vi "Balancing Controller.vi"(6 "Configuration":T1={"Accelerometer Bias"={"X (m/s)"=0.0, "Y (m/s)"=0.0, "Z (m/s)"=0.0}, "Gyroscope Bias"={"X (m/s)"=0.0, "Y (m/s)"=0.0, "Z (m/s)"=0.0}, "Steering Motor Gear Ratio"=611.0, "Steering Pully Gear Ratio"=1.0, "Steering Encoder CPR"=500.0, "Steering Motor Max RPM"=4000.0, "Wheelbase (m)"=1.12, "Fork Angle (rad)"=1.3, "Balancing Controller"={"Kp (/s)"=1.0, "Kd (1)"=1.0}, "Max Allowed Steering Angle (rad)"=0.7, "Task Periods"={"Emergency Stop (us)"=10000, "IMU (us)"=10000, "Steering Motor Encoder (us)"=10000, "State Estimator (us)"=10000, "Balancing Controller (us)"=10000, "GNSS (us)"=10000, "Logging (us)"=50000, "Drive Motor (us)"=100000}, "Drive Motor Gear Ratio"=0.7, "lr"=0.4964, "lf"=0.5986, "lambda"=1.2217, "k1"=0.004472, "k2"=0.09678, "e1_max"=11.331, "Ad_t"=0.95971, "Bd_t"=0.01, "C_t"=2.20588, "D_t"=0.0, "Wheel radius"=0.311}, 8 "Measurement In":refnum<data-value>, 9 "State Estimate In":refnum<data-value>, 10 "Trajectory In":refnum<data-value>, 11 "Error In":errorcluster) -> (0 "Measurement Out":refnum<data-value>, 1 "State Estimate Out":refnum<data-value>, 3 "Error Out":errorcluster, 4 "Steering Angle Rate (rad/s)":dbl, 5 "Input balancing":dbl)   [LabVIEW 2021]
uses:
  State Estimator/State Estimate.ctl
  State Estimator/Measurements.ctl
  IMU/IMU Data.ctl
  Steering Motor Encoder/Steering Motor Encoder Data.ctl
  GNSS/GNSS Data.ctl
  Trajectory Control/Trajectory_Control.ctl
  Configuration/Configuration.ctl
  Logging/Log Level.ctl
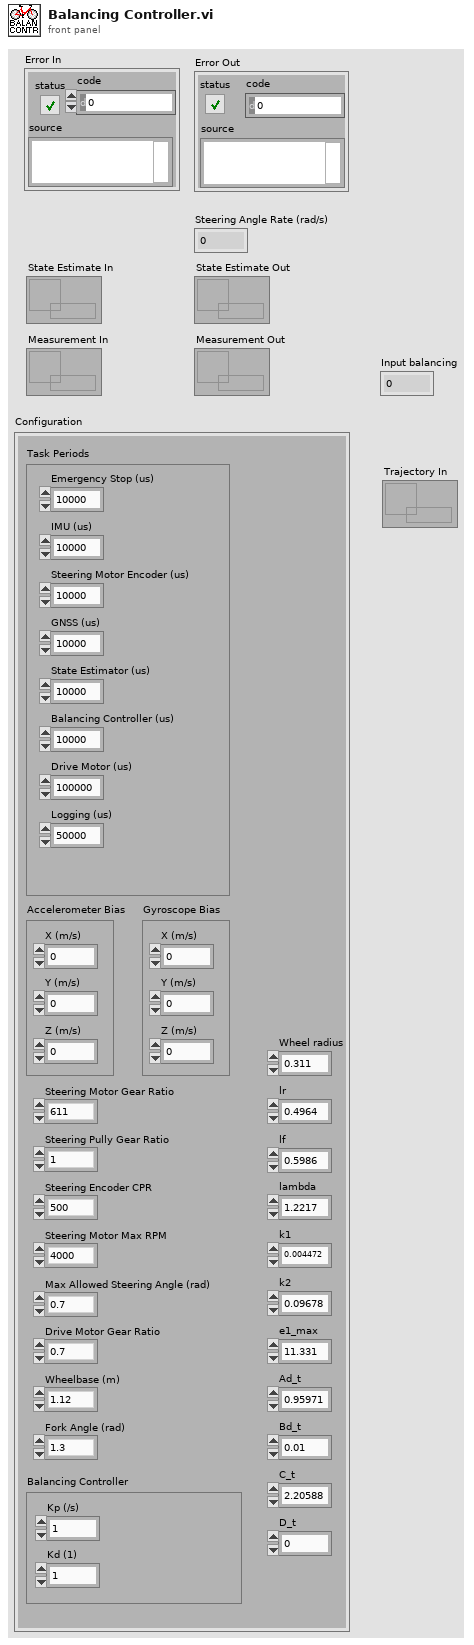
[diagram p1: front panel]
types:
  T1 = typedef "Configuration.ctl" = cluster{"Accelerometer Bias":cluster{"X (m/s)":dbl, "Y (m/s)":dbl, "Z (m/s)":dbl}, "Gyroscope Bias":cluster{"X (m/s)":dbl, "Y (m/s)":dbl, "Z (m/s)":dbl}, "Steering Motor Gear Ratio":dbl, "Steering Pully Gear Ratio":dbl, "Steering Encoder CPR":dbl, "Steering Motor Max RPM":dbl, "Wheelbase (m)":dbl, "Fork Angle (rad)":dbl, "Balancing Controller":cluster{"Kp (/s)":dbl, "Kd (1)":dbl}, "Max Allowed Steering Angle (rad)":dbl, "Task Periods":cluster{"Emergency Stop (us)":i64, "IMU (us)":i64, "Steering Motor Encoder (us)":i64, "State Estimator (us)":i64, "Balancing Controller (us)":i64, "GNSS (us)":i64, "Logging (us)":i64, "Drive Motor (us)":i64}, "Drive Motor Gear Ratio":dbl, "lr":dbl, "lf":dbl, "lambda":dbl, "k1":dbl, "k2":dbl, "e1_max":dbl, "Ad_t":dbl, "Bd_t":dbl, "C_t":dbl, "D_t":dbl, "Wheel radius":dbl}
  T2 = typedef "Log Level.ctl" = enum16{"Error", "Warning", "Info"}
  T3 = typedef "Trajectory_Control.ctl" = cluster{"Rollref":dbl, "Closestpoint":dbl, "Error1":dbl, "Error2":dbl, "Dpsiref_cont":dbl, "Lateral_cont":dbl, "Heading_cont":dbl, "Reset_traj":dbl, "Iteration":dbl}
  T4 = typedef "State Estimate.ctl" = cluster{"X (m)":dbl, "Y (m)":dbl, "Psi (rad)":dbl, "Roll (rad)":dbl, "Roll Rate (rad/s)":dbl, "delta":dbl, "velocity":dbl, "Iterations":dbl}
  T5 = typedef "Measurements.ctl" = cluster{"IMU Data":T6, "Steering Motor Encoder Data":T7, "GNSS Data":T8}
  T6 = typedef "IMU Data.ctl" = cluster{"Gyroscope":cluster{"X (rad/s)":dbl, "Y (rad/s)":dbl, "Z (rad/s)":dbl}, "Accelerometer":cluster{"X (m/s^2)":dbl, "Y (m/s^2)":dbl, "Z (m/s^2)":dbl}, "Flag IMU":dbl}
  T7 = typedef "Steering Motor Encoder Data.ctl" = cluster{"Encoder Position (counts)":i32, "Steering Angle (rad)":dbl, "Flag Steering Encoder":dbl}
  T8 = typedef "GNSS Data.ctl" = cluster{"Latitude (rad)":dbl, "Longitude (rad)":dbl, "Altitude (m)":dbl, "Speed (m/s)":dbl, "Heading (rad)":dbl, "Fix Quality":i32, "Number of Satellites":i32, "Latitude (deg)":dbl, "Longitude (deg)":dbl, "Flag GNSS":dbl}
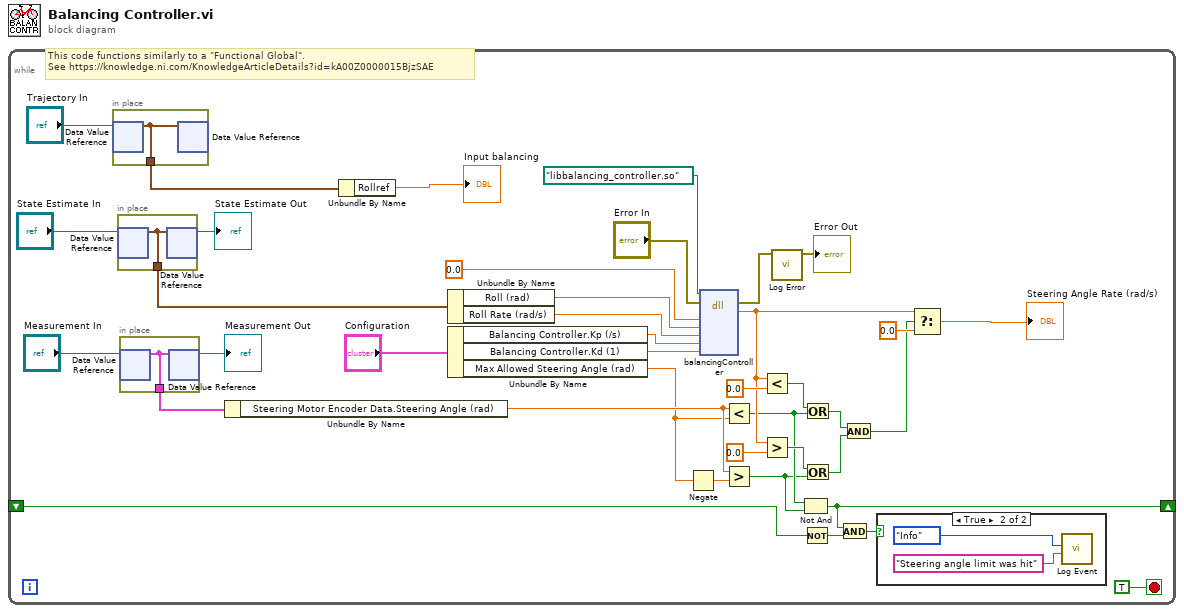
[diagram p0: block diagram]
diagram:
  # "This code functions similarly to a \"Functional Global\".\nSee https://knowledge.ni.com/KnowledgeArticleDetails?id=kA00Z0000015BjzSAE"
  n1 = while {
    shift-right: [w10] -> _
    shift-left: _ -> [w12]
    stop <- TRUE stop-if-true
    n2 = in-place {
      in-place-border: [w40] -> w6
      n3 = in-place-dvr #1 ("Data Value Reference Read / Write Element")("Trajectory In") -> (w40:T3)  [unwired: 1 out]
      n4 = in-place-dvr #1(w40) -> ()  [unwired: 2 out]
    }
    n5 = in-place {
      in-place-border: [w44] -> w33
      n6 = in-place-dvr #2("State Estimate In") -> (w44:T4)  [unwired: 1 out]
      n7 = in-place-dvr #2(w44) -> (→"State Estimate Out":refnum<data-value>)  [unwired: 1 out]
    }
    n8 = in-place {
      in-place-border: [w43] -> w30
      n9 = in-place-dvr #3("Measurement In") -> (w43:T5)  [unwired: 1 out]
      n10 = in-place-dvr #3(w43) -> (→"Measurement Out":refnum<data-value>)  [unwired: 1 out]
    }
    n11 = Unbundle By Name(w30) -> ("Steering Motor Encoder Data.Steering Angle (rad)"=w18:dbl)
    n12 = Unbundle By Name(w6) -> ("Rollref"=→"Input balancing":dbl)
    n13 = Unbundle By Name(w33) -> ("Roll (rad)"=w1:dbl, "Roll Rate (rad/s)"=w2:dbl)
    n14 = Unbundle By Name("Configuration") -> ("Balancing Controller.Kp (/s)"=w36:dbl, "Balancing Controller.Kd (1)"=w35:dbl, "Max Allowed Steering Angle (rad)"=w17:dbl)
    n15 = Negate(x=w17) -> (-x=w19:dbl)
    n16 = dll-call lib="?" fn="balancingController"(path in=path "libbalancing_controller.so", error in="Error In", "rollReference"=0.0, "roll"=w1, "rollRate"=w2, "Kp"=w36, "Kd"=w35) -> (error out=w15:errorcluster, "Steering Angle Rate"=w23:dbl)  [unwired: 6 in, 1 out]
    n17 = Less?(x=w18, y=w17) -> (x < y?=w9:bool)
    n18 = Greater?(x=w18, y=w19) -> (0:w8:bool)
    n19 = Less?(x=w23, y=0.0) -> (x < y?=w26:bool)
    n20 = Greater?(x=w23, y=0.0) -> (0:w22:bool)
    n21 = call "Log Error.vi"("Error In"=w15) -> ("Error Out"=→"Error Out":errorcluster)  [unwired: 10 in]
    n22 = Not And(1:w8, 2:w9) -> (0:w10:bool)
    n23 = Not(x=w12) -> (.not. x?=w13:bool)
    n24 = Or(x=w26, y=w9) -> (x .or. y?=w25:bool)
    n25 = Or(x=w22, y=w8) -> (x .or. y?=w21:bool)
    n26 = And(x=w10, y=w13) -> (x .and. y?=w11:bool)
    n27 = And(x=w25, y=w21) -> (x .and. y?=w20:bool)
    n28 = case shown="True" w11 {
      frame False {
      }
      frame True {
        n29 = call "Log Event.vi"("Message"="Steering angle limit was hit", "Log Level"=Log_Level."Info") -> ()  [unwired: 9 in, 1 out]
      }
    }
    n30 = Select(t=w23, s=w20, f=0.0) -> (s? t:f=→"Steering Angle Rate (rad/s)":dbl)
  }
